vi "Open Log File.vi"(8 "error in (no error)":errorcluster, 11 "Log File Specification in":refnum<class "Log File Specification.lvclass">) -> (0 "error out":errorcluster, 1 "Instance File Path":path, 2 "Log File out":refnum<class "Log File.lvclass">, 3 "Log File Specification out":refnum<class "Log File Specification.lvclass">)   [LabVIEW 2015, in "Waveform Data Logger Shared.lvlib" / "Log File Specification.lvclass"]
doc: "Builds an instance file path and opens a new file instance using that path."
uses:
  Log File Specification.lvclass
  Engine/Classes/Logs/Log Files/Log File/Log File.lvclass
  Log File Specification.lvclass/Log File Specification.ctl
  Utility/Format File Path for Linux.vi
  <vilib>/Utility/libraryn.llb/Get File Extension.vi
  <vilib>/Utility/error.llb/Error Cluster From Error Code.vi
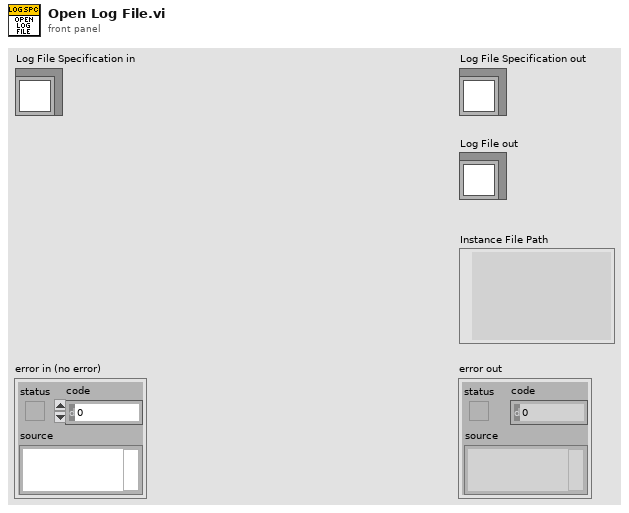
[diagram p1: front panel]
types:
  T1 = typedef "Waveform Data Logger Engine.lvlib/Log File.lvclass/Operation.ctl" = enum16{"open", "open or create", "create or replace", "create", "open (read-only)"}
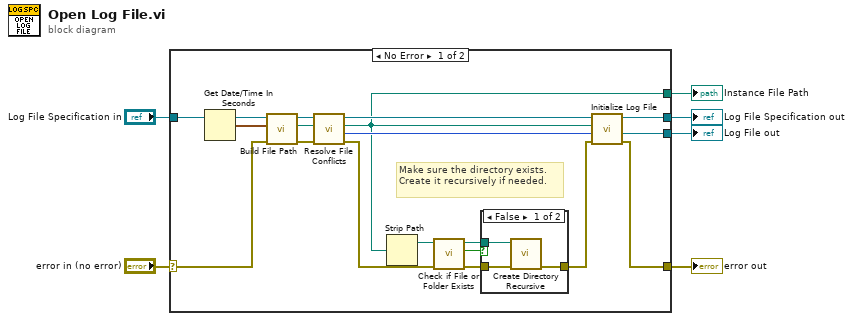
[diagram p0: block diagram]
diagram:
  n1 = case shown="No Error" "error in (no error)" {
    selector: "error in (no error)" -> [w24 w30]
    tunnel: [w13 w30] -> w5
    tunnel: [w22 w29] -> w3
    tunnel: "Log File Specification in" -> [w20 w29]
    tunnel: [w21 _] -> w2
    tunnel: [w14 _] -> w1
    frame No Error {
      # "Make sure the directory exists. Create it recursively if needed."
      n2 = Get Date/Time In Seconds() -> (seconds since 1Jan1904=w23:timestamp)
      n3 = call "Build File Path.vi"("error in (no error)"=w24, "Time Stamp"=w23, "Log File Specification in"=w20) -> ("error out"=w19:errorcluster, "Instance File Path"=w15:path, "Log File Specification out"=w18:refnum<class "Log File Specification.lvclass">)  [unwired: 6 in]
      n4 = call "Resolve File Conflicts.vi"("error in (no error)"=w19, "Instance File Path in"=w15, "Log File Specification in"=w18) -> ("error out"=w9:errorcluster, "Operation"=w16:T1, "Instance File Path out"=w14:path, "Log File Specification out"=w17:refnum<class "Log File Specification.lvclass">)  [unwired: 5 in]
      n5 = Strip Path(path=w14) -> (stripped path=w10:path)  [unwired: 1 out]
      n6 = call <vilib>:"Check if File or Folder Exists.vi"("error in (no error)"=w9, "path"=w10) -> ("error out"=w12:errorcluster, "file or folder exists?"=w7:bool, "dup path"=w11:path)  [unwired: 7 in]
      n7 = case shown="False" w7 {
        tunnel: w12 -> [w27 w28]
        tunnel: w11 -> [w26 _]
        tunnel: [w25 w28] -> w8
        frame False {
          n8 = call <vilib>:"Create Directory Recursive.vi"("error in (no error)"=w27, "directory"=w26) -> ("error out"=w25:errorcluster)  [unwired: 3 in, 2 out]
        }
        frame True {
        }
      }
      n9 = call "Initialize Log File.vi"("error in (no error)"=w8, "Operation"=w16, "File Path"=w14, "Log File Specification in"=w17) -> ("error out"=w13:errorcluster, "Log File out"=w21:refnum<class "Log File.lvclass">, "Log File Specification out"=w22:refnum<class "Log File Specification.lvclass">)  [unwired: 5 in]
    }
    frame Error {
    }
  }
  "error out" <- w5
  "Log File Specification out" <- w3
  "Log File out" <- w2
  "Instance File Path" <- w1
